vi "InitializeSubVI.vi"(0 "Exposure Time (secs)":sgl format="%.2f") -> (1 "Camera Status:":bool, 2 "Initialize (bool 1)":bool, 3 "Set image (bool 2)":bool, 4 "Check timings (bool 3)":bool)   [LabVIEW 2018]
uses:
  atmcd32d.dll
panel:
  in  "Tab Control":T1(tab)
  in  "Trigger":u32(ring) items=["Internal", "External"]
  out "Initialize":u32
  out "Calculated Exposure Value":sgl format="%.5f"
  out "Detector X Pixels":i32
  out "Check Timings":u32
  out "Set Acquisition Mode":u32
  out "Set Readout Mode":u32
  out "Set Trigger Mode":u32
  out "Set Exposure Time":u32
  out "Get Detector":u32
  out "Detector Y Pixels":i32
  out "Set Gate Mode":u32
  out "Set Image":u32
  # "Status"
  # "Return values"
  # "USB iStarIMAG32at.VI"
  # "Acquisition Mode: Single Scan\nReadout Mode: Full Resolution Image"
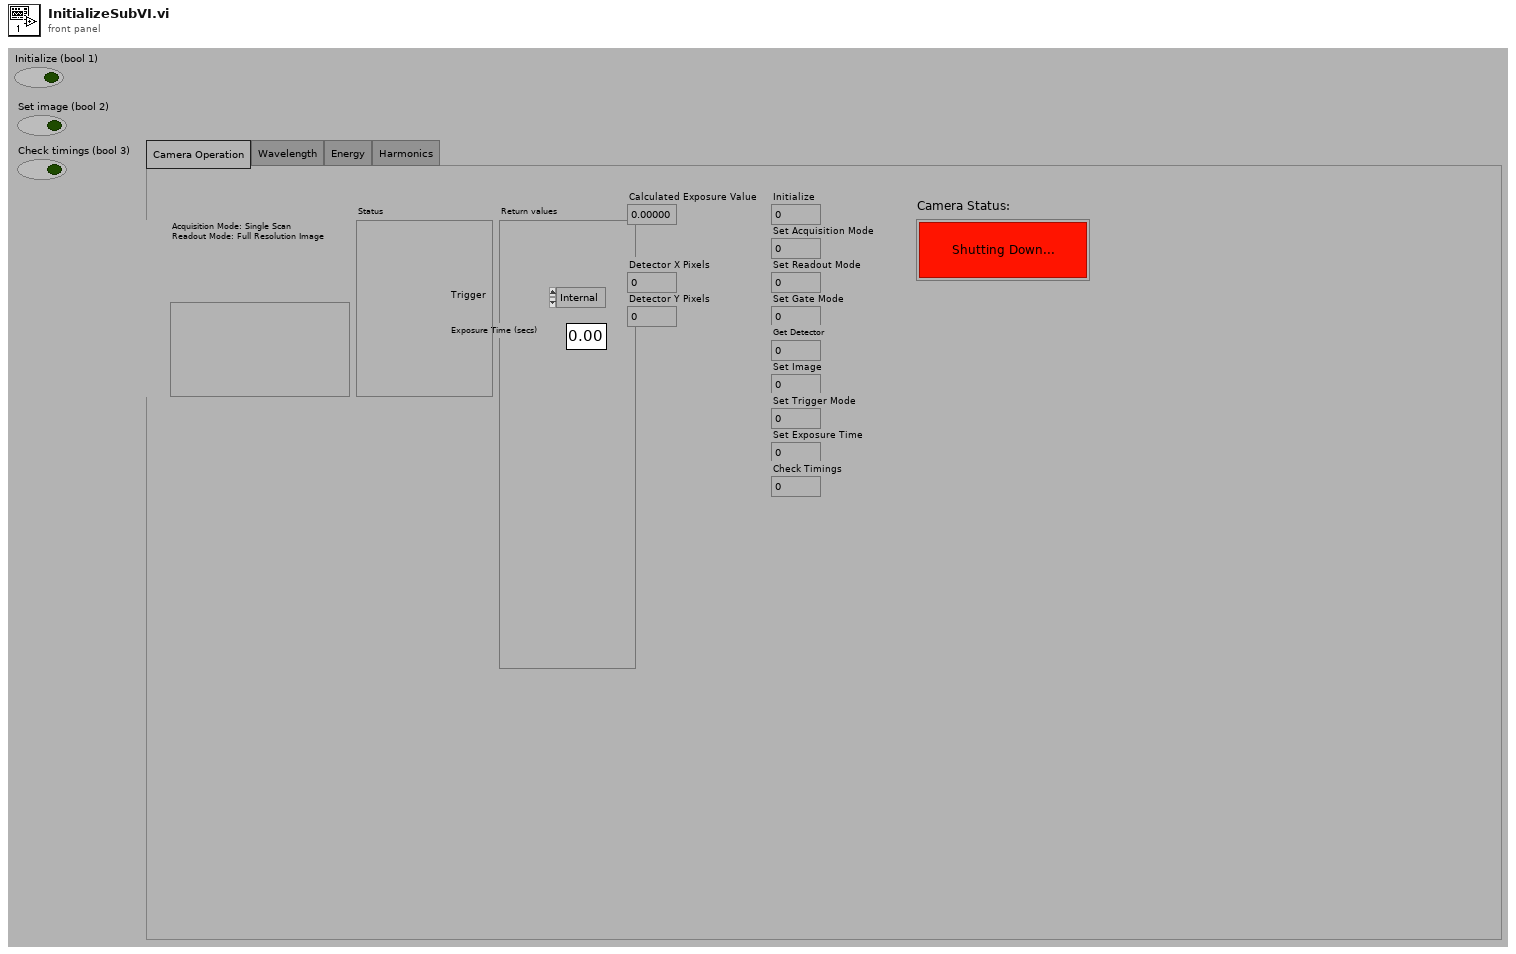
[diagram p1: front panel]
types:
  T1 = enum32{"Camera Operation", "Wavelength", "Energy", "Harmonics"}
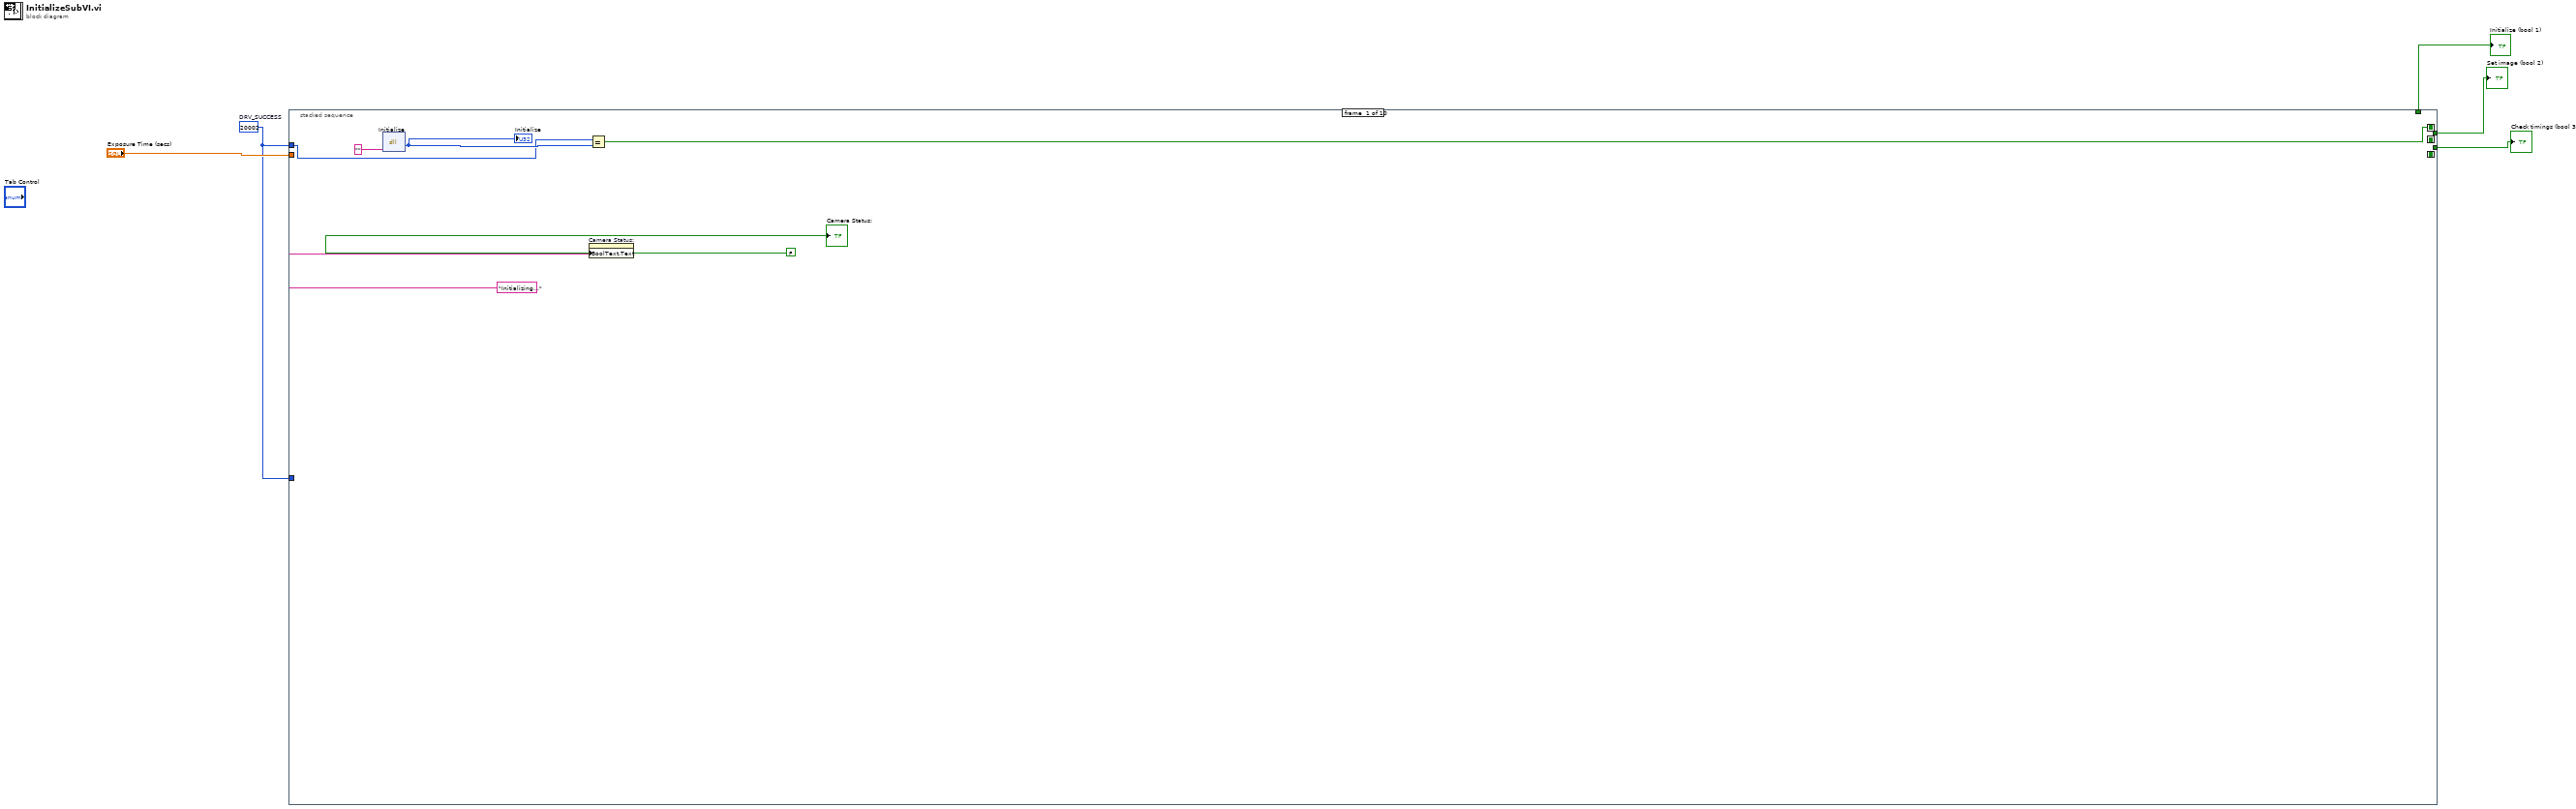
[diagram p0: block diagram]
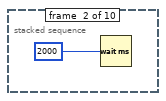
[diagram p2: hidden frame]
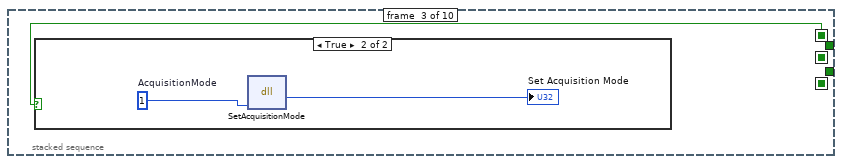
[diagram p3: hidden frame]
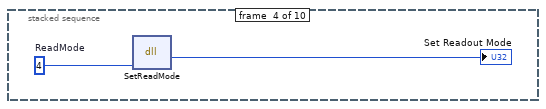
[diagram p5: hidden frame]
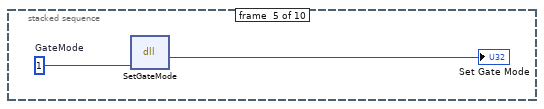
[diagram p6: hidden frame]
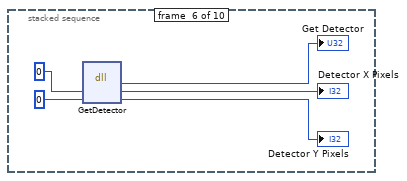
[diagram p7: hidden frame]
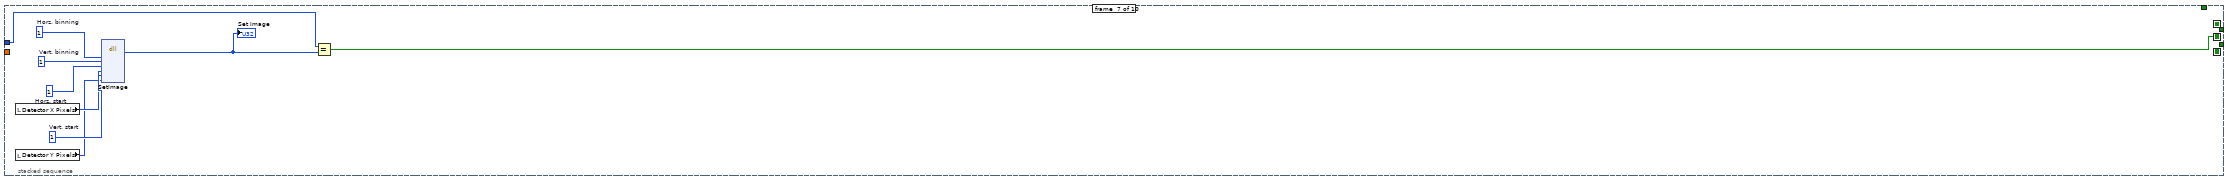
[diagram p8: hidden frame]
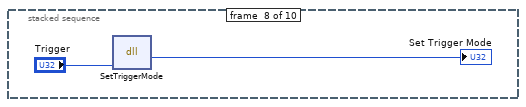
[diagram p9: hidden frame]
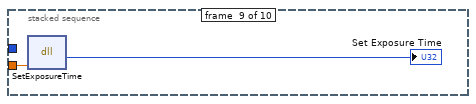
[diagram p10: hidden frame]
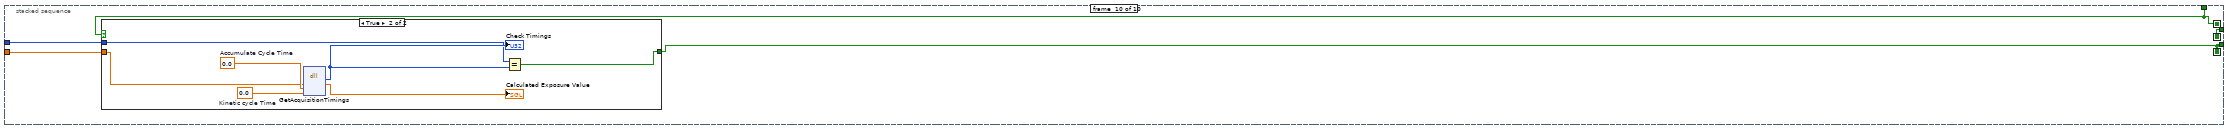
[diagram p11: hidden frame]
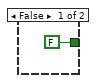
[diagram p12: hidden frame]
diagram:
  w4 = 20002  # DRV_SUCCESS
  n1 = stacked-sequence {
    seq-local: [w9 _ _ _ _ _ _ _ _ _] -> [_ _ w13 _ _ _ _ _ _ w38]
    seq-local: [_ _ _ _ _ _ _ _ _ w40] -> [_ _ _ _ _ _ _ _ _ _]
    seq-local: [_ _ _ _ _ _ w25 _ _ _] -> [_ _ _ _ _ _ _ _ _ w39]
    tunnel: "Exposure Time (secs)" -> [_ _ _ _ _ _ _ _ w37 w42]
    tunnel: w4 -> [w10 _ _ _ _ _ w27 _ _ w41]
    tunnel: w4 -> [_ _ _ _ _ _ _ _ _ _]
    tunnel: [_ _ _ _ _ _ _ _ _ w40] -> w3
    tunnel: [_ _ _ _ _ _ _ _ _ w39] -> w2
    tunnel: [_ _ _ _ _ _ _ _ _ w38] -> w1
    frame #0 {
      n2 = dll-call lib="atmcd32d.dll" fn="Initialize" label="Call Library Function Initialize"("") -> (w11:u32)  [unwired: 4 in, 2 out]
      "Initialize" <- w11
      n3 = property on="Camera Status:" class="Bool (strict)"("BoolText.Text"="Initializing..." ("String")) -> ()  [unwired: 2 in, 2 out]
      n4 = Equal?(x=w10, y=w11) -> (x = y?=w9:bool)
      "Camera Status:" <- FALSE ("Camera Status:")
    }
    frame #1 {
      n5 = Wait (ms)(milliseconds to wait=u32 2000) -> ()  [unwired: 1 out]
    }
    frame #2 {
      n6 = case shown="True" w13 {
        frame False {
        }
        frame True {
          w15 = u16 1  # AcquisitionMode
          n7 = dll-call lib="atmcd32d.dll" fn="SetAcquisitionMode" label="Call Library Function SetAcquisitionMode"(w15) -> (→"Set Acquisition Mode":u32)  [unwired: 4 in, 2 out]
        }
      }
    }
    frame #3 {
      w17 = u16 4  # ReadMode
      n8 = dll-call lib="atmcd32d.dll" fn="SetReadMode" label="Call Library Function SetReadMode"(w17) -> (→"Set Readout Mode":u32)  [unwired: 4 in, 2 out]
    }
    frame #4 {
      w19 = u16 1  # GateMode
      n9 = dll-call lib="atmcd32d.dll" fn="SetGateMode" label="Call Library Function SetGateMode"(w19) -> (→"Set Gate Mode":u32)  [unwired: 4 in, 2 out]
    }
    frame #5 {
      n10 = dll-call lib="atmcd32d.dll" fn="GetDetector" label="Call Library FunctionGetDetector"(i16 0, i16 0) -> (→"Get Detector":u32, →"Detector X Pixels":i32, →"Detector Y Pixels":i32)  [unwired: 3 in, 2 out]
    }
    frame #6 {
      w30 = u16 1  # Vert. start
      w31 = u16 1  # Horz. start
      w32 = u16 1  # Vert. binning
      w33 = u16 1  # Horz. binning
      n11 = local read "Detector X Pixels"() -> (w29:i32)
      n12 = local read "Detector Y Pixels"() -> (w28:i32)
      n13 = dll-call lib="atmcd32d.dll" fn="SetImage" label="Call Library Function SetImage"(w33, w32, w31, w29, w30, w28) -> (w26:u32)  [unwired: 9 in, 2 out]
      "Set Image" <- w26
      n14 = Equal?(x=w27, y=w26) -> (x = y?=w25:bool)
    }
    frame #7 {
      n15 = dll-call lib="atmcd32d.dll" fn="SetTriggerMode" label="Call Library Function SetTrigger Mode"("Trigger") -> (→"Set Trigger Mode":u32)  [unwired: 4 in, 2 out]
    }
    frame #8 {
      n16 = dll-call lib="atmcd32d.dll" fn="SetExposureTime" label="Call Library FunctionSet Exposure Time"(w37) -> (→"Set Exposure Time":u32)  [unwired: 4 in, 2 out]
    }
    frame #9 {
      n17 = case shown="True" w38 {
        tunnel: w42 -> [_ w47]
        tunnel: w41 -> [_ w44]
        tunnel: [FALSE w46] -> w40
        frame False {
        }
        frame True {
          w49 = sgl 0.0  # Accumulate Cycle Time
          w50 = sgl 0.0  # Kinetic cycle Time
          n18 = dll-call lib="atmcd32d.dll" fn="GetAcquisitionTimings" label="Call Library Function Check Timings"(w47, w49, w50) -> (w45:u32, →"Calculated Exposure Value":sgl)  [unwired: 5 in, 2 out]
          "Check Timings" <- w45
          n19 = Equal?(x=w44, y=w45) -> (x = y?=w46:bool)
        }
      }
    }
  }
  "Set image (bool 2)" <- w2
  "Check timings (bool 3)" <- w3
  "Initialize (bool 1)" <- w1
